vi "Get_AxisArray_FromConf.vi"(8 "error in (no error)":errorcluster, 11 "MotionModule runtime in":refnum<class "MotionModule runtime.lvclass">) -> (0 "error out":errorcluster, 2 "AxisArray_FromConf":string[](array[string]), 3 "MotionModule runtime out":refnum<class "MotionModule runtime.lvclass">)   [LabVIEW 2017, in "MotionModule runtime.lvclass"]
uses:
  MotionModule runtime.lvclass
  MotionModule runtime.lvclass/MotionModule runtime.ctl
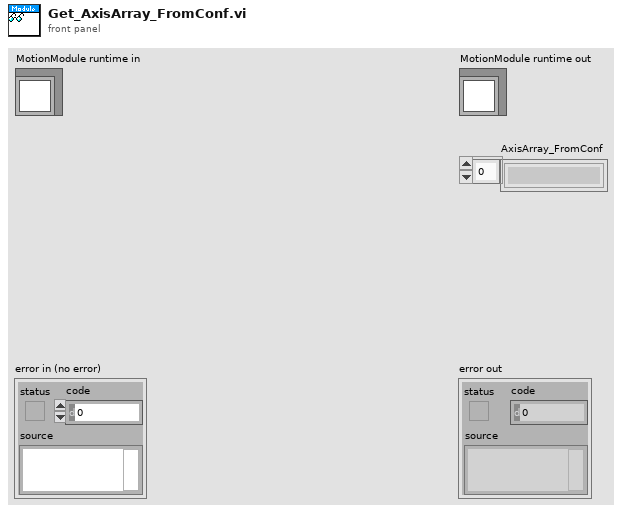
[diagram p1: front panel]
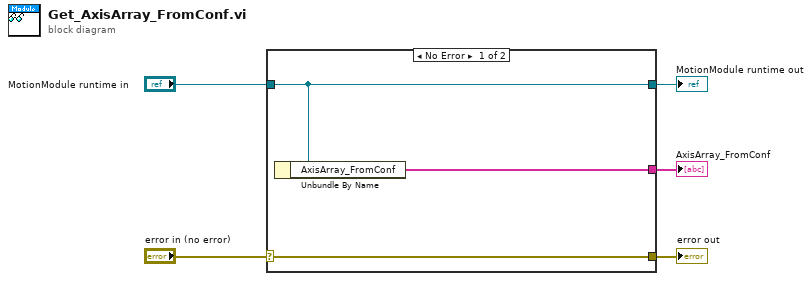
[diagram p0: block diagram]
diagram:
  n1 = case shown="No Error" "error in (no error)" {
    selector: "error in (no error)" -> [w8 w9]
    tunnel: [w8 w9] -> w4
    tunnel: [w7 w10] -> w2
    tunnel: "MotionModule runtime in" -> [w7 w10]
    tunnel: [w6 _] -> w1
    frame No Error {
      n2 = Unbundle By Name(w7) -> ("AxisArray_FromConf"=w6:string[])
    }
    frame Error {
    }
  }
  "error out" <- w4
  "MotionModule runtime out" <- w2
  "AxisArray_FromConf" <- w1
